vi "Compute Waveform.vi"(4 "% duty cycle\n(square wave only, 50)":dbl=50.0, 6 "Period":dbl=100.0 format="%.2f", 7 "phase (0 deg)":dbl format="%.2f", 8 "offset (0.0)":dbl format="%.2f", 9 "amplitude (1.0)":dbl=1.0 format="%.2f", 10 "number of points (1000)":i32=1000, 11 "signal type (0:sine)":u16(ring) items=["Sine Wave", "Square Wave", "Sawtooth", "Triangle Wave"]) -> (3 "output waveform":dbl[](array[numeric]) format="%.2f")   [LabVIEW 2009]
doc: "This is a subVI used by the function generator analog output example.\n\nThis VI computes a single cycle of a waveform - square, sine, triangle or sawtooth with the number of points, amplitude, offset and phase specified. The single output waveform is put into a transposed 2D array so that it can be fed directly into the AO Write VI.\n\nNote: for multiple channel waveform generation, the output should be modified as a 1D array so that multiple waveforms can be strung together with an array builder VI."
panel:
  out "waveform graph":ext[](graph)
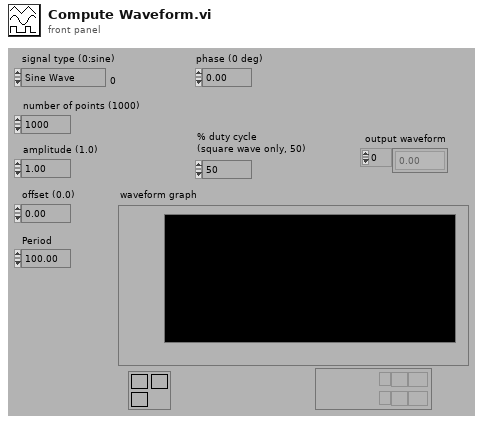
[diagram p1: front panel]
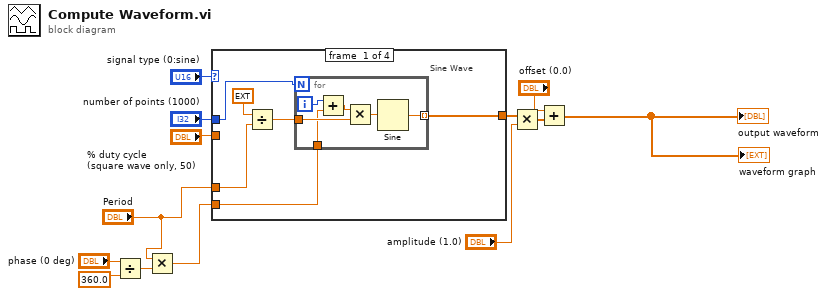
[diagram p0: block diagram]
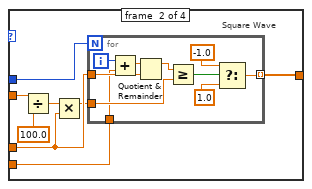
[diagram p2: hidden frame]
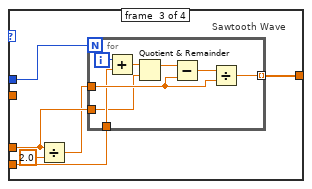
[diagram p3: hidden frame]
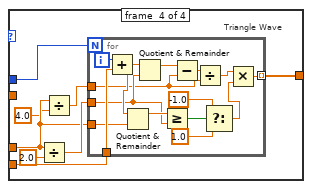
[diagram p4: hidden frame]
diagram:
  n1 = Divide(x="phase (0 deg)", y=360.0) -> (x/y=w5:dbl)
  n2 = Multiply(x="Period", y=w5) -> (x*y=w2:dbl)
  n3 = case shown="3.." "signal type (0:sine)" {
    tunnel: "number of points (1000)" -> [w17 w33 w49 w65]
    tunnel: [w16 w30 w48 w64] -> w11
    tunnel: "% duty cycle\n(square wave only, 50)" -> [_ w32 _ _]
    tunnel: "Period" -> [w15 w27 w45 w60]
    tunnel: w2 -> [w14 w29 w47 w63]
    frame #0 {
      # "Sine Wave"
      n4 = Divide(x=ext 6.283185307179586477, y=w15) -> (x/y=w18:ext)
      n5 = for {
        N: w17 -> [_]
        tunnel: w18 -> [w24]
        tunnel: [w23] -> w16 mode=indexing
        tunnel: w14 -> [w20]
        i -> [w21]
        n6 = Add(x=w21, y=w20) -> (x+y=w22:dbl)
        n7 = Multiply(x=w22, y=w24) -> (x*y=w25:ext)
        n8 = Sine(x=w25) -> (sin(x)=w23:ext)
      }
    }
    frame #1 {
      # "Square Wave"
      n9 = Divide(x=w32, y=100.0) -> (x/y=w28:dbl)
      n10 = Multiply(x=w28, y=w27) -> (x*y=w26:dbl)
      n11 = for {
        N: w33 -> [_]
        tunnel: w27 -> [w43]
        tunnel: w26 -> [w39]
        tunnel: [w38] -> w30 mode=indexing
        tunnel: w29 -> [w34]
        i -> [w35]
        n12 = Add(x=w35, y=w34) -> (x+y=w36:dbl)
        n13 = Quotient & Remainder(x=w36, y=w43) -> (x-y*floor(x/y)=w37:dbl)  [unwired: 1 out]
        n14 = Greater Or Equal?(x=w37, y=w39) -> (x >= y?=w40:bool)
        n15 = Select(t=-1.0, s=w40, f=1.0) -> (s? t:f=w38:dbl)
      }
    }
    frame #2 {
      # "Sawtooth Wave"
      n16 = Divide(x=w45, y=2.0) -> (x/y=w44:dbl)
      n17 = for {
        N: w49 -> [_]
        tunnel: [w57] -> w48 mode=indexing
        tunnel: w44 -> [w55]
        tunnel: w47 -> [w53]
        tunnel: w45 -> [w51]
        i -> [w54]
        n18 = Add(x=w54, y=w53) -> (x+y=w52:dbl)
        n19 = Quotient & Remainder(x=w52, y=w51) -> (x-y*floor(x/y)=w50:dbl)  [unwired: 1 out]
        n20 = Subtract(x=w50, y=w55) -> (x-y=w56:dbl)
        n21 = Divide(x=w56, y=w55) -> (x/y=w57:dbl)
      }
    }
    frame #3 {
      # "Triangle Wave"
      n22 = Divide(x=w60, y=2.0) -> (x/y=w61:dbl)
      n23 = Divide(x=w60, y=4.0) -> (x/y=w58:dbl)
      n24 = for {
        N: w65 -> [_]
        tunnel: [w75] -> w64 mode=indexing
        tunnel: w61 -> [w71]
        tunnel: w63 -> [w78]
        tunnel: w60 -> [w73]
        tunnel: w58 -> [w66]
        i -> [w79]
        n25 = Add(x=w79, y=w78) -> (x+y=w74:dbl)
        n26 = Quotient & Remainder(x=w74, y=w73) -> (x-y*floor(x/y)=w72:dbl)  [unwired: 1 out]
        n27 = Quotient & Remainder(x=w74, y=w71) -> (x-y*floor(x/y)=w77:dbl)  [unwired: 1 out]
        n28 = Greater Or Equal?(x=w72, y=w71) -> (x >= y?=w70:bool)
        n29 = Subtract(x=w77, y=w66) -> (x-y=w80:dbl)
        n30 = Divide(x=w80, y=w66) -> (x/y=w76:dbl)
        n31 = Select(t=-1.0, s=w70, f=1.0) -> (s? t:f=w67:dbl)
        n32 = Multiply(x=w76, y=w67) -> (x*y=w75:dbl)
      }
    }
  }
  n33 = Multiply(x=w11, y="amplitude (1.0)") -> (x*y=w9:ext[])
  n34 = Add(x="offset (0.0)", y=w9) -> (x+y=→"output waveform" →"waveform graph":ext[])
